vi "poziomy.vi"(3 "pauza":bool, 4 "Akcja":enum16{"Przygotuj listę", "Sprawdź"}(ring)) -> (0 "KONIEC":bool, 1 "Aktualny stan":T1)   [LabVIEW 2014]
uses:
  main_states.ctl
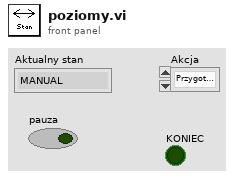
[diagram p1: front panel]
types:
  T1 = typedef "main_states.ctl" = enum16{"MANUAL", "REWIND", "FORWARD", "OFF"}
  T2 = cluster{"Cluster":cluster{"Stan poziomy":T1, "Czas":dbl}}[]
  T3 = cluster{"Cluster":cluster{"Stan poziomy":T1, "Czas":dbl}}
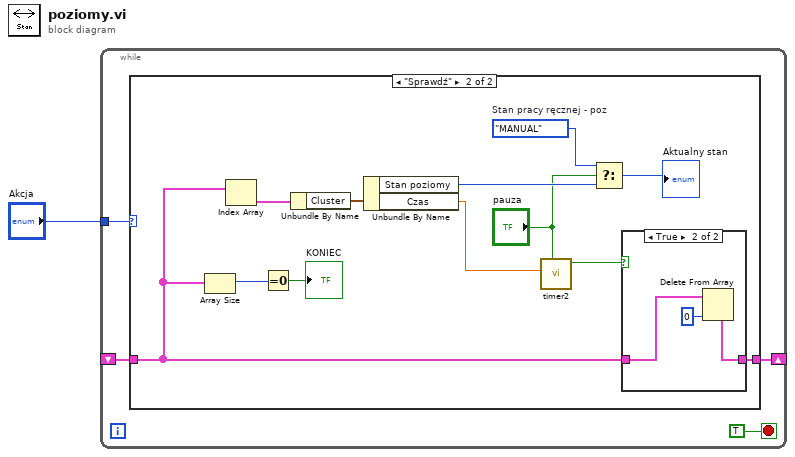
[diagram p0: block diagram]
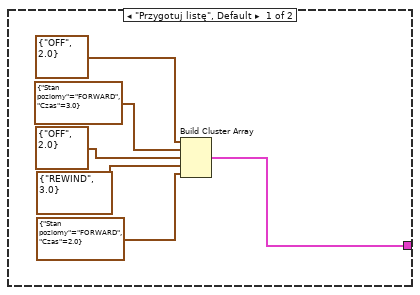
[diagram p2: hidden frame]
diagram:
  n1 = while {
    shift-right: [w3] -> _
    shift-left: _ -> [w4]
    tunnel: "Akcja" -> [w2]
    stop <- TRUE stop-if-true
    n2 = case shown="\"Sprawdź\"" w2 {
      tunnel: w4 -> [_ w14]
      tunnel: [w7 w21] -> w3
      frame "Przygotuj listę", Default {
        n3 = Build Cluster Array(cluster{"Stan poziomy":T1, "Czas":dbl} {"Stan poziomy"=enum."OFF", "Czas"=2.0} ("Cluster"), cluster{"Stan poziomy":T1, "Czas":dbl} {"Stan poziomy"=enum."FORWARD", "Czas"=3.0} ("Cluster"), cluster{"Stan poziomy":T1, "Czas":dbl} {"Stan poziomy"=enum."OFF", "Czas"=2.0} ("Cluster"), cluster{"Stan poziomy":T1, "Czas":dbl} {"Stan poziomy"=enum."REWIND", "Czas"=3.0} ("Cluster"), cluster{"Stan poziomy":T1, "Czas":dbl} {"Stan poziomy"=enum."FORWARD", "Czas"=2.0} ("Cluster")) -> (w7:T2)
      }
      frame "Sprawdź" {
        w19 = main_states."MANUAL"  # Stan pracy ręcznej - poz
        n4 = Array Size(array=w14) -> (size(s)=w13:i32)
        n5 = Index Array(array=w14) -> (element=w22:T3)  [unwired: 1 in]
        n6 = Equal To 0?(x=w13) -> (x = 0?=→"KONIEC":bool)
        n7 = Unbundle By Name(w22) -> ("Cluster"=w23:cluster{"Stan poziomy":T1, "Czas":dbl})
        n8 = Unbundle By Name(w23) -> ("Stan poziomy"=w20:T1, "Czas"=w17:dbl)
        n9 = call "timer2.vi"("pauza"="pauza", "Czas"=w17) -> ("czy czas upłynął"=w15:bool)  [unwired: 9 in]
        n10 = Select(t=w19, s="pauza", f=w20) -> (s? t:f=→"Aktualny stan":T1)
        n11 = case shown="True" w15 {
          tunnel: [w24 w27] -> w21
          tunnel: w14 -> [w24 w25]
          frame False {
          }
          frame True {
            n12 = Delete From Array(array=w25, index=0) -> (array with subset deleted=w27:T2)  [unwired: 1 in, 1 out]
          }
        }
      }
    }
  }
